vi "Address Space Size.vi"(2 "DIO":refnum<class "Digital IO.lvclass">) -> (6 "size":u32)   [LabVIEW 2017, in "Digital IO.lvlib" / "Digital IO.lvclass"]
uses:
  Digital IO.lvclass
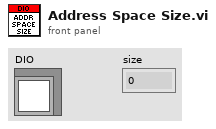
[diagram p1: front panel]
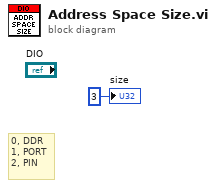
[diagram p0: block diagram]
diagram:
  # "0, DDR\n1, PORT\n2, PIN"
  "size" <- u32 3 ("size")
